vi "DRIVE_STRAIGHT_NAVX_RAMPARTS.vi"(10 "argv":string[](array[string]), 11 "args":u8) -> ()   [LabVIEW 2015]
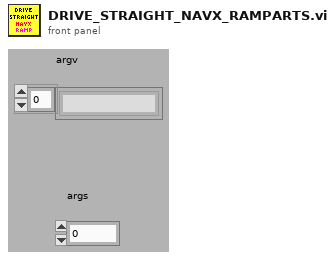
[diagram p1: front panel]
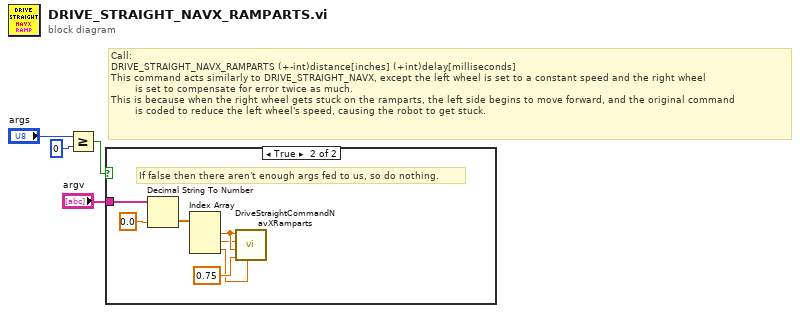
[diagram p0: block diagram]
diagram:
  # "Call:\nDRIVE_STRAIGHT_NAVX_RAMPARTS (+-int)distance[inches] (+int)delay[milliseconds]\nThis command acts similarly to DRIVE_STRAIGHT_NAVX, except the left wheel is set to a constant speed and the right wheel\n        is set to compensate for error twice as much.\nThis is because when the right wheel gets stuck on the ramparts, the left side begins to move forward, and the original command\n        is coded to reduce the left wheel's speed, causing the robot to get stuck."
  n1 = Greater Or Equal?(x="args", y=u8 0) -> (x >= y?=w4:bool)
  n2 = case shown="True" w4 {
    tunnel: "argv" -> [_ w11]
    frame False {
    }
    frame True {
      # "If false then there aren't enough args fed to us, so do nothing."
      n3 = Decimal String To Number(string=w11, default (0L)=0.0 ("default (0 I32)")) -> (number=w8:dbl[])  [unwired: 2 out]
      n4 = Index Array(array=w8) -> (element #1=w7:dbl, element #2=w6:dbl, element #3=w5:dbl)  [unwired: 3 in]
      n5 = call "DriveStraightCommandNavXRamparts.vi"("TONDelay"=w5, "speed"=0.75, "Fwd Bwd"=w7, "Delay ms"=w6, "distance"=w7) -> ()  [unwired: 7 in]
    }
  }
